vi "dilutionCalcR.vi"(0 "Clust Refnum":refnum<vi>) -> ()   [LabVIEW 2011]
uses:
  source_noDilute.ctl
  source_noDilution.ctl
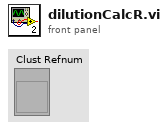
[diagram p1: front panel]
types:
  T1 = typedef "source_noDilute.ctl" = cluster{"Dilution":bool, "Calculated":u16, "MFC1 flow":dbl, "MFC2 flow":dbl, "MFC3 flow":dbl, "Bubbler (main)":T2}
  T2 = typedef "source_noDilution.ctl" = cluster{"Flow":dbl, "Prep":bool, "Run":bool, "Active":bool}
  T3 = enum8{"Enabled", "Disabled", "Disabled and Grayed Out"}
  T4 = cluster{"Controls[][0]":refnum<vi>, "Controls[][1]":refnum<vi>, "Controls[][2]":refnum<vi>, "Controls[][3]":refnum<vi>, "Controls[][4]":refnum<vi>, "Controls[][5]":refnum<vi>, "Controls[][6]":refnum<vi>, "Controls[][7]":refnum<vi>, "Controls[][8]":refnum<vi>}
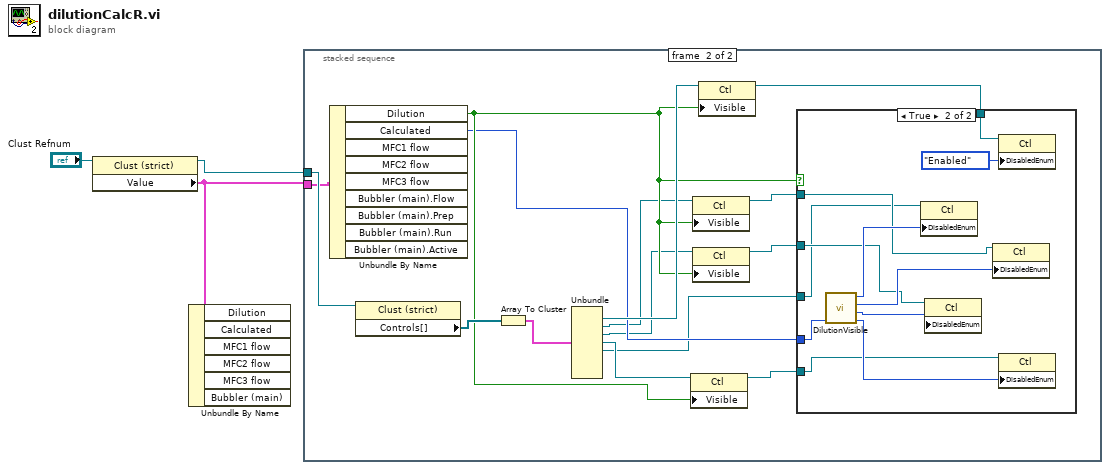
[diagram p0: block diagram]
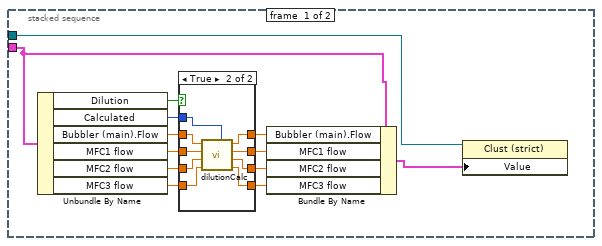
[diagram p2: hidden frame]
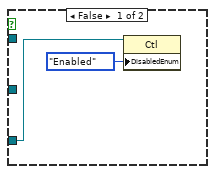
[diagram p4: hidden frame]
diagram:
  n1 = property class="Clust (strict)"(reference="Clust Refnum") -> (reference out=w2:refnum<vi>, "Value"=w1:T1)  [unwired: 1 in, 1 out]
  n2 = Unbundle By Name(w1) -> ()  [unwired: 6 out]
  n3 = stacked-sequence {
    tunnel: w2 -> [w4 w44]
    tunnel: w1 -> [w6 w36]
    frame #0 {
      n4 = Unbundle By Name(w6) -> ("Dilution"=w16:bool, "Calculated"=w15:u16, "Bubbler (main).Flow"=w12:dbl, "MFC1 flow"=w13:dbl, "MFC2 flow"=w14:dbl, "MFC3 flow"=w11:dbl)
      n5 = case shown="True" w16 {
        tunnel: w15 -> [_ w29]
        tunnel: w14 -> [w18 w26]
        tunnel: w13 -> [w19 w27]
        tunnel: w12 -> [w20 w28]
        tunnel: w11 -> [w17 w25]
        tunnel: [w20 w24] -> w10
        tunnel: [w19 w23] -> w9
        tunnel: [w18 w22] -> w8
        tunnel: [w17 w21] -> w7
        frame False {
        }
        frame True {
          n6 = call "dilutionCalc.vi"("Calculated"=w29, "MFC3"=w25, "MFC2"=w26, "MFC1"=w27, "flow"=w28) -> ("MFC3 out"=w21:dbl, "MFC2 out"=w22:dbl, "MFC1 out"=w23:dbl, "flow out"=w24:dbl)  [unwired: 1 in]
        }
      }
      n7 = Bundle By Name(cluster=w6, "Bubbler (main).Flow"=w10, "MFC1 flow"=w9, "MFC2 flow"=w8, "MFC3 flow"=w7) -> (w5:T1)
      n8 = property class="Clust (strict)"(reference=w4, "Value"=w5) -> ()  [unwired: 1 in, 2 out]
    }
    frame #1 {
      n9 = Unbundle By Name(w36) -> ("Dilution"=w40:bool, "Calculated"=w39:u16)  [unwired: 7 out]
      n10 = property class="Clust (strict)"(reference=w44) -> ("Controls[]"=w43:refnum<vi>[])  [unwired: 1 in, 2 out]
      n11 = Array To Cluster(array=w43) -> (cluster=w42:T4)
      n12 = Unbundle(w42) -> ("Controls[][1]"=w41:refnum<vi>, "Controls[][2]"=w35:refnum<vi>, "Controls[][3]"=w34:refnum<vi>, "Controls[][4]"=w33:refnum<vi>, "Controls[][5]"=w30:refnum<vi>)  [unwired: 4 out]
      n13 = property class="Ctl"(reference=w33, "Visible"=w40) -> (reference out=w32:refnum<vi>)  [unwired: 1 in, 1 out]
      n14 = property class="Ctl"(reference=w35, "Visible"=w40) -> (reference out=w37:refnum<vi>)  [unwired: 1 in, 1 out]
      n15 = property class="Ctl"(reference=w34, "Visible"=w40) -> (reference out=w38:refnum<vi>)  [unwired: 1 in, 1 out]
      n16 = property class="Ctl"(reference=w41, "Visible"=w40) -> (reference out=w31:refnum<vi>)  [unwired: 1 in, 1 out]
      n17 = case shown="True" w40 {
        tunnel: w39 -> [_ w57]
        tunnel: w30 -> [w46 w49]
        tunnel: w38 -> [_ w51]
        tunnel: w37 -> [_ w50]
        tunnel: w32 -> [_ w52]
        tunnel: w31 -> [_ w48]
        frame False {
          n18 = property class="Ctl"(reference=w46, "DisabledEnum"=T3."Enabled" ("Disabled")) -> ()  [unwired: 1 in, 2 out]
        }
        frame True {
          n19 = call "DilutionVisible.vi"("calculated"=w57) -> ("MFC3"=w53:u16, "MFC2"=w54:u16, "MFC1"=w55:u16, "flow"=w56:u16)  [unwired: 3 in]
          n20 = property class="Ctl"(reference=w49, "DisabledEnum"=w56) -> ()  [unwired: 1 in, 2 out]
          n21 = property class="Ctl"(reference=w51, "DisabledEnum"=w54) -> ()  [unwired: 1 in, 2 out]
          n22 = property class="Ctl"(reference=w50, "DisabledEnum"=w55) -> ()  [unwired: 1 in, 2 out]
          n23 = property class="Ctl"(reference=w48, "DisabledEnum"=T3."Enabled" ("Disabled")) -> ()  [unwired: 1 in, 2 out]
          n24 = property class="Ctl"(reference=w52, "DisabledEnum"=w53) -> ()  [unwired: 1 in, 2 out]
        }
      }
    }
  }
